vi "Requests from uServices.vi"(8 "error in (no error)":errorcluster, 9 "Data":variant, 10 "Requests":T1, 11 "Guardian in":refnum<class "Guardian.lvclass">) -> (0 "error out":errorcluster, 3 "Guardian out":refnum<class "Guardian.lvclass">)   [LabVIEW 2026, in "TALOS.lvlib" / "Guardian.lvlib" / "Guardian.lvclass"]
uses:
  Guardian.lvclass
  C:/LabVIEW Code/TALOS/talos/Ancestor/Ancestor/Ancestor.lvclass
  C:/LabVIEW Code/TALOS/builds/Actor Framework PPL/Actor Framework.lvlibp/1abvi3w/vi.lib/ActorFramework/Actor/Actor.lvclass
  Requests.ctl
  Ancestor/Ancestor/Ancestor.lvclass/Ancestor.ctl
  Guardian Messages/Broadcast to Guardians Msg/Broadcast to Guardians Msg.lvclass/Broadcast to Guardians Msg.ctl
  Guardian.lvclass/Guardian.ctl
  Guardian Messages/Message to uService Msg/Message to uService Msg.lvclass/Message to uService Msg.ctl
  <vilib>/Utility/error.llb/Trim Whitespace (string).vi
  Ancestor/Ancestor/Read ID.vi
  <vilib>/Utility/error.llb/Trim Whitespace One-Sided.vi
  Support VIs/Generate Error.vi
  FGV/Error Memory/Get Error Description.vi
  Support VIs/Get PC name.vi
  Support VIs/Get Class Name.vi
  <vilib>/Utility/error.llb/Clear Errors.vi
  FGV/Error Memory/Error Memory Core.vi
  <vilib>/AdvancedString/Delimited String to 1D String Array.vi
  <vilib>/AdvancedString/Delimited String to 1D String Array (string).vi
  Support VIs/Circus Root Path.vi
  FGV/Error Memory/Error Crt Lvl checker.vi
  FGV/Error Memory/Error Memory Core.vi/40c8088d-b597-4017-91af-faa98e00292e.vi
  FGV/Error Memory/Error Memory Core.vi/d4a3ab98-063c-4e44-b43d-fbdcfe6c2be2.vi
  Support VIs/Global Memory.vi
  <vilib>/Utility/LVClass/Get LV Class Name.vi
  Support VIs/Is in Packed Library.vi
  Support VIs/TALOS Root path.vi
  Support VIs/Read CSV worksheet.vi
  Support VIs/Global Constants.vi
  <vilib>/Utility/error.llb/General Error Handler.vi
  <vilib>/Utility/config.llb/Open Config Data.vi
  <vilib>/Utility/config.llb/Get Section Names.vi
  <vilib>/Utility/config.llb/Get Key Names.vi
  <vilib>/Utility/config.llb/Read Key.vi
  <vilib>/Utility/config.llb/Read Key (String).vi
  <vilib>/Utility/config.llb/Close Config Data.vi
  builds/Actor Framework PPL/Actor Framework.lvlibp/1abvi3w/vi.lib/ActorFramework/Message Enqueuer/Enqueue.vi
  Support VIs/Error Log.vi
  Ancestor/Ancestor/Ancestor.lvclass
  <vilib>/Comparison/Equal/Equal Functor/Equal Functor.lvclass
  Guardian Messages/Broadcast to Guardians Msg/Broadcast to Guardians Msg.lvclass
  Guardian Messages/Message to uService Msg/Message to uService Msg.lvclass
  builds/Actor Framework PPL/Actor Framework.lvlibp/1abvi3w/vi.lib/ActorFramework/Actor/Actor.lvclass
  TALOS.lvlib
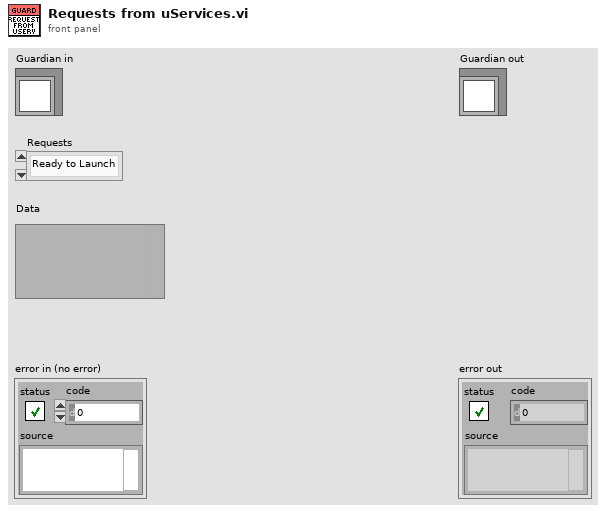
[diagram p1: front panel]
types:
  T1 = typedef "TALOS.lvlib/Guardian.lvlib/Guardian.lvclass/Requests.ctl" = enum16{"Ready to Launch", "Start RUN", "Stop RUN", "Update DAQ Params", "Update Error Listbox", "Update Run Status", "Update Kasli Log", "Run Stopped with Errors", "Switch uS View", "Dismiss All Errors"}
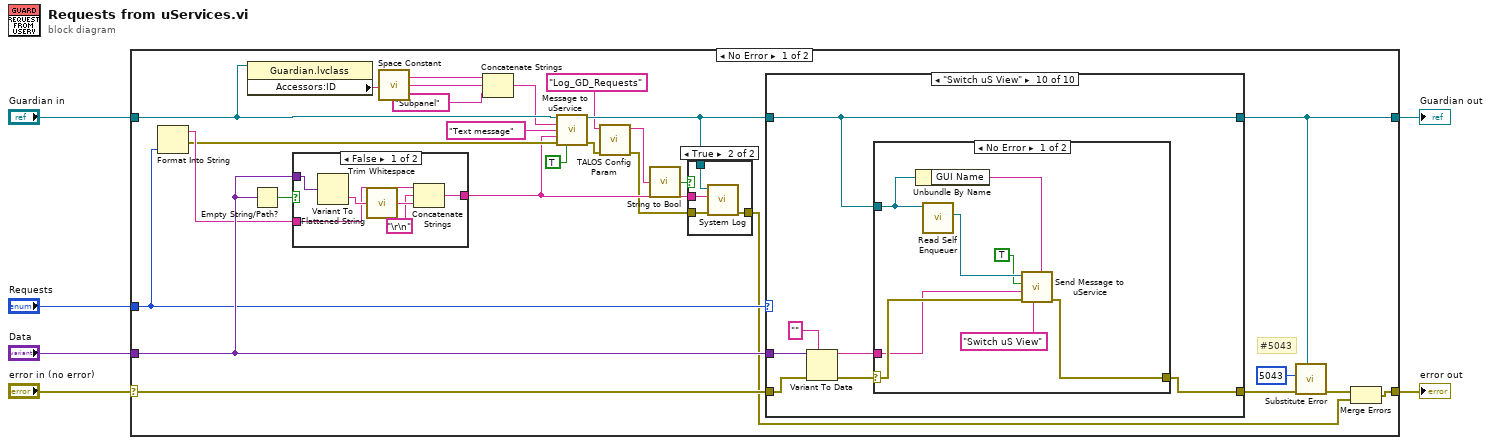
[diagram p0: block diagram]
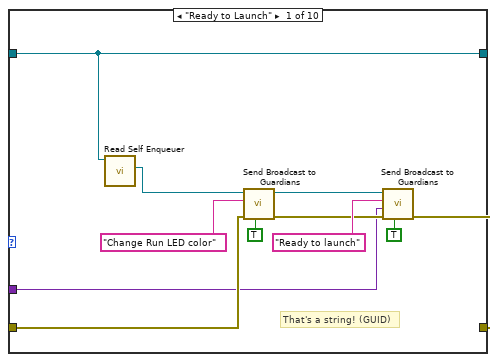
[diagram p4: hidden frame]
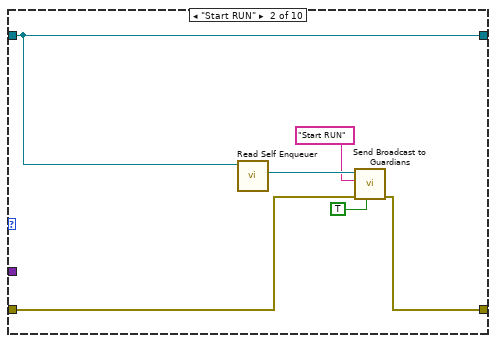
[diagram p5: hidden frame]
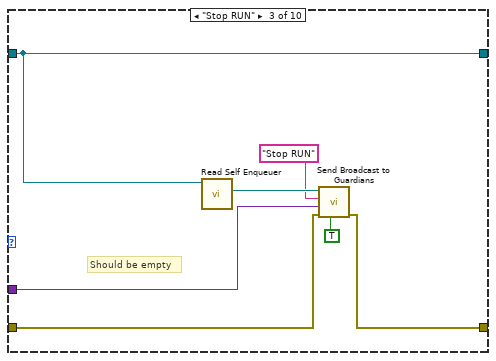
[diagram p6: hidden frame]
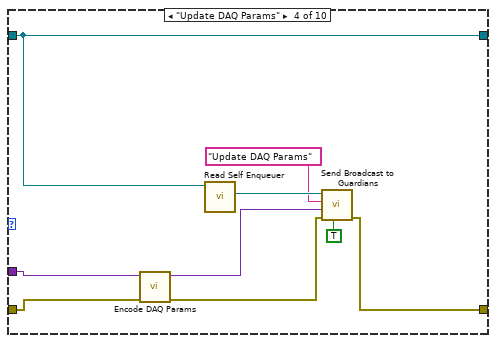
[diagram p7: hidden frame]
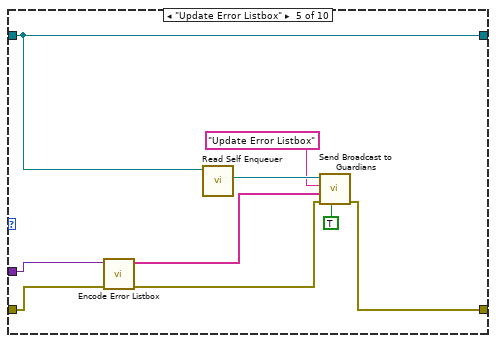
[diagram p8: hidden frame]
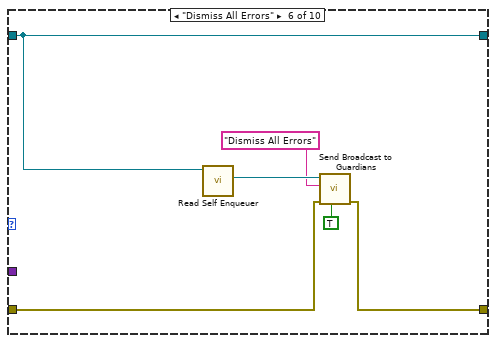
[diagram p9: hidden frame]
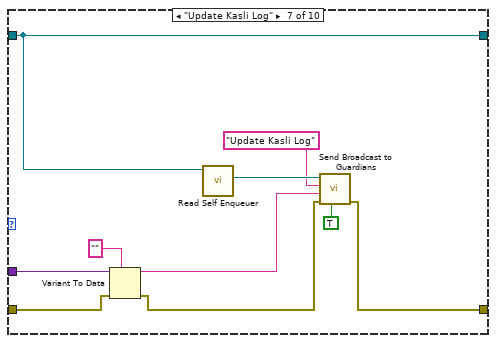
[diagram p10: hidden frame]
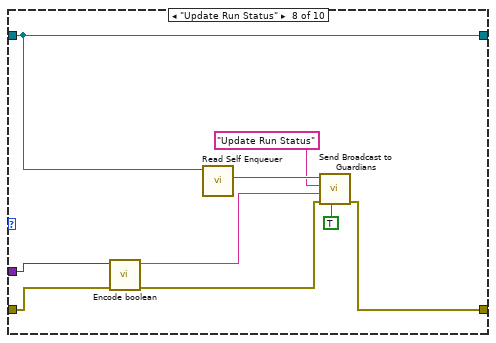
[diagram p11: hidden frame]
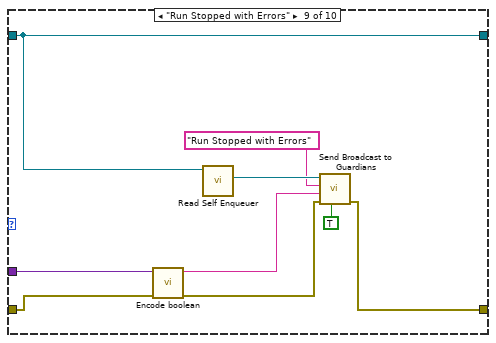
[diagram p12: hidden frame]
diagram:
  n1 = case shown="No Error" "error in (no error)" {
    selector: "error in (no error)" -> [w32 w138]
    tunnel: [w27 w138] -> w5
    tunnel: [w8 w137] -> w3
    tunnel: "Guardian in" -> [w21 w137]
    tunnel: "Requests" -> [w29 _]
    tunnel: "Data" -> [w30 _]
    frame No Error {
      # "#5043"
      n2 = Format Into String(w29) -> (resulting string=w28:string, error out=w24:errorcluster)  [unwired: 3 in]
      n3 = property class="Guardian.lvclass"(reference=w21) -> ("Accessors:ID"=w20:string)  [unwired: 1 in, 2 out]
      n4 = Empty String/Path?(string/path=w30) -> (empty?=w31:bool)
      n5 = case shown="False" w31 {
        tunnel: [w40 w44] -> w23
        tunnel: w30 -> [w39 _]
        tunnel: w28 -> [w38 w44]
        frame False {
          n6 = Variant To Flattened String(Variant=w39) -> (data string=w43:string)  [unwired: 1 out]
          n7 = call-poly <vilib>:"Trim Whitespace.vi"("string"=w43) -> ("trimmed string"=w42:string)  [unwired: 1 in]
          n8 = Concatenate Strings(w38, "\r\n", w42) -> (w40:string)
        }
        frame True {
        }
      }
      n9 = call <vilib>:"Space Constant.vi"() -> ("String"=w17:string)
      n10 = Concatenate Strings(w20, w17, "Subpanel" ("uService ID")) -> (w19:string)
      n11 = call "Message to uService.vi"("Guardian in"=w21, "uService ID"=w19, "Message"="Text message", "Data"=w23, "error in (no error)"=w24, "Locale?"=TRUE) -> ("Guardian out"=w16:refnum<class "Guardian.lvclass">, "error out"=w11:errorcluster)  [unwired: 8 in]
      n12 = call "TALOS Config Param.vi"("error in (no error)"=w11, "Parameter Name"="Log_GD_Requests") -> ("error out"=w12:errorcluster, "Output"=w13:string)  [unwired: 8 in]
      n13 = call "String to Bool.vi"("String"=w13) -> ("Boolean"=w15:bool)
      n14 = case shown="True" w15 {
        tunnel: [w33 w37] -> w26
        tunnel: w23 -> [_ w36]
        tunnel: w16 -> [_ w35]
        tunnel: w12 -> [w33 w34]
        frame False {
        }
        frame True {
          n15 = call "System Log.vi"("error in (no error)"=w34, "Text to log"=w36, "Object in"=w35) -> ("error out"=w37:errorcluster)  [unwired: 8 in]
        }
      }
      n16 = case shown="\"Switch uS View\"" w29 {
        tunnel: w16 -> [w55 w59 w65 w75 w86 w92 w100 w109 w118 w121]
        tunnel: [w55 w59 w65 w75 w86 w92 w100 w109 w118 w121] -> w8
        tunnel: w32 -> [w47 w57 w68 w70 w80 w90 w95 w105 w114 w126]
        tunnel: w30 -> [w45 _ w63 w72 w79 _ w98 w106 w115 w127]
        tunnel: [w53 w58 w64 w74 w85 w91 w99 w108 w117 w122] -> w10
        frame "Ready to Launch" {
          # "That's a string! (GUID)"
          n17 = call "Read Self Enqueuer.vi"("Actor"=w55) -> ("Self Enqueuer"=w46:refnum<class "Message Enqueuer.lvclass">)  [unwired: 10 in]
          n18 = call "Send Broadcast to Guardians.vi"("Local also?"=TRUE, "error in (no error)"=w47, "Message"="Change Run LED color", "Message Enqueuer"=w46) -> ("error out"=w48:errorcluster, "Message Enqueuer out"=w49:refnum<class "Message Enqueuer.lvclass">)  [unwired: 6 in]
          n19 = call "Send Broadcast to Guardians.vi"("Local also?"=TRUE, "error in (no error)"=w48, "Data"=w45, "Message"="Ready to launch", "Message Enqueuer"=w49) -> ("error out"=w53:errorcluster)  [unwired: 5 in, 1 out]
        }
        frame "Start RUN" {
          n20 = call "Read Self Enqueuer.vi"("Actor"=w59) -> ("Self Enqueuer"=w61:refnum<class "Message Enqueuer.lvclass">)  [unwired: 10 in]
          n21 = call "Send Broadcast to Guardians.vi"("Local also?"=TRUE, "error in (no error)"=w57, "Message"="Start RUN", "Message Enqueuer"=w61) -> ("error out"=w58:errorcluster)  [unwired: 6 in, 1 out]
        }
        frame "Stop RUN" {
          # "Should be empty"
          n22 = call "Read Self Enqueuer.vi"("Actor"=w65) -> ("Self Enqueuer"=w67:refnum<class "Message Enqueuer.lvclass">)  [unwired: 10 in]
          n23 = call "Send Broadcast to Guardians.vi"("Local also?"=TRUE, "error in (no error)"=w68, "Data"=w63, "Message"="Stop RUN", "Message Enqueuer"=w67) -> ("error out"=w64:errorcluster)  [unwired: 5 in, 1 out]
        }
        frame "Update DAQ Params" {
          n24 = call "Encode DAQ Params.vi"("error in (no error)"=w70, "Data in"=w72) -> ("error out"=w71:errorcluster, "Data out"=w69:variant)  [unwired: 8 in]
          n25 = call "Read Self Enqueuer.vi"("Actor"=w75) -> ("Self Enqueuer"=w77:refnum<class "Message Enqueuer.lvclass">)  [unwired: 10 in]
          n26 = call "Send Broadcast to Guardians.vi"("Local also?"=TRUE, "error in (no error)"=w71, "Data"=w69, "Message"="Update DAQ Params", "Message Enqueuer"=w77) -> ("error out"=w74:errorcluster)  [unwired: 5 in, 1 out]
        }
        frame "Update Error Listbox" {
          n27 = call "Encode Error Listbox.vi"("error in (no error)"=w80, "Data"=w79) -> ("error out"=w81:errorcluster, "Encoded Msg"=w78:string[])  [unwired: 8 in]
          n28 = call "Read Self Enqueuer.vi"("Actor"=w86) -> ("Self Enqueuer"=w84:refnum<class "Message Enqueuer.lvclass">)  [unwired: 10 in]
          n29 = call "Send Broadcast to Guardians.vi"("Local also?"=TRUE, "error in (no error)"=w81, "Data"=w78, "Message"="Update Error Listbox", "Message Enqueuer"=w84) -> ("error out"=w85:errorcluster)  [unwired: 5 in, 1 out]
        }
        frame "Dismiss All Errors" {
          n30 = call "Read Self Enqueuer.vi"("Actor"=w92) -> ("Self Enqueuer"=w89:refnum<class "Message Enqueuer.lvclass">)  [unwired: 10 in]
          n31 = call "Send Broadcast to Guardians.vi"("Local also?"=TRUE, "error in (no error)"=w90, "Message"="Dismiss All Errors", "Message Enqueuer"=w89) -> ("error out"=w91:errorcluster)  [unwired: 6 in, 1 out]
        }
        frame "Update Kasli Log" {
          n32 = Variant To Data(error in=w95, type="", Variant=w98) -> (data=w93:string, error out=w96:errorcluster)
          n33 = call "Read Self Enqueuer.vi"("Actor"=w100) -> ("Self Enqueuer"=w102:refnum<class "Message Enqueuer.lvclass">)  [unwired: 10 in]
          n34 = call "Send Broadcast to Guardians.vi"("Local also?"=TRUE, "error in (no error)"=w96, "Data"=w93, "Message"="Update Kasli Log", "Message Enqueuer"=w102) -> ("error out"=w99:errorcluster)  [unwired: 5 in, 1 out]
        }
        frame "Update Run Status" {
          n35 = call "Encode boolean.vi"("error in (no error)"=w105, "Data"=w106) -> ("error out"=w103:errorcluster, "String"=w104:string)  [unwired: 8 in]
          n36 = call "Read Self Enqueuer.vi"("Actor"=w109) -> ("Self Enqueuer"=w111:refnum<class "Message Enqueuer.lvclass">)  [unwired: 10 in]
          n37 = call "Send Broadcast to Guardians.vi"("Local also?"=TRUE, "error in (no error)"=w103, "Data"=w104, "Message"="Update Run Status", "Message Enqueuer"=w111) -> ("error out"=w108:errorcluster)  [unwired: 5 in, 1 out]
        }
        frame "Run Stopped with Errors" {
          n38 = call "Encode boolean.vi"("error in (no error)"=w114, "Data"=w115) -> ("error out"=w112:errorcluster, "String"=w113:string)  [unwired: 8 in]
          n39 = call "Read Self Enqueuer.vi"("Actor"=w118) -> ("Self Enqueuer"=w120:refnum<class "Message Enqueuer.lvclass">)  [unwired: 10 in]
          n40 = call "Send Broadcast to Guardians.vi"("Local also?"=TRUE, "error in (no error)"=w112, "Data"=w113, "Message"="Run Stopped with Errors", "Message Enqueuer"=w120) -> ("error out"=w117:errorcluster)  [unwired: 5 in, 1 out]
        }
        frame "Switch uS View" {
          n41 = Variant To Data(error in=w126, type="", Variant=w127) -> (data=w123:string, error out=w124:errorcluster)
          n42 = case shown="No Error" w124 {
            selector: w124 -> [w134 w136]
            tunnel: w123 -> [w131 _]
            tunnel: [w133 w136] -> w122
            tunnel: w121 -> [w130 _]
            frame No Error {
              n43 = Unbundle By Name(w130) -> ("GUI Name"=w129:string)
              n44 = call "Read Self Enqueuer.vi"("Actor"=w130) -> ("Self Enqueuer"=w135:refnum<class "Message Enqueuer.lvclass">)  [unwired: 10 in]
              n45 = call "Send Message to uService.vi"("uService ID"=w129, "Message"="Switch uS View", "error in (no error)"=w134, "Data"=w131, "Locale?"=TRUE, "Message Enqueuer"=w135) -> ("error out"=w133:errorcluster)  [unwired: 4 in, 1 out]
            }
            frame Error {
            }
          }
        }
      }
      n46 = call "Substitute Error.vi"("LabVIEW Object"=w8, "error in (no error)"=w10, "Error Code"=5043) -> ("error out"=w9:errorcluster)  [unwired: 8 in]
      n47 = Merge Errors(w9, w26) -> (w27:errorcluster)
    }
    frame Error {
    }
  }
  "error out" <- w5
  "Guardian out" <- w3
